vi "addDefectiveRows.vi"(0 "reference in":refnum<class "excelFile.lvclass">, 5 "error in (no error)":errorcluster) -> (14 "reference out":refnum<class "excelFile.lvclass">, 19 "error out":errorcluster)   [LabVIEW 2016, in "excelFile.lvclass"]
uses:
  excelFile.lvclass
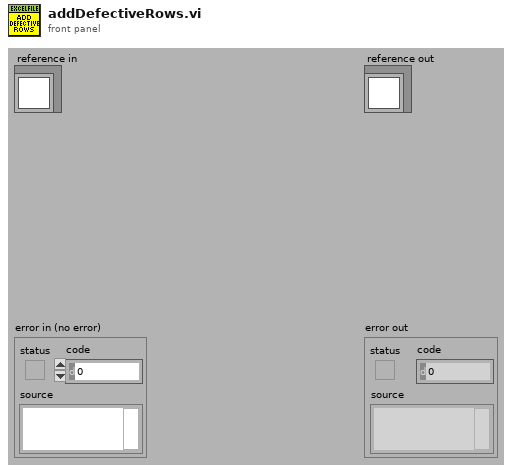
[diagram p1: front panel]
types:
  T1 = typedef "excelFile.lvclass/ObjectAttributesRef.ctl" = refnum<data-value>
  T2 = typedef "excelFile.lvclass/ObjectAttributes.ctl" = cluster{"MyAttribute":dbl, "path":string, "Refnum Excel":cluster{"Excel._Application":refnum<k7>, "Workbooks":refnum<k7>, "Open":refnum<k7>}, "data":string[][][], "save":bool, "fileType":T3, "rowsColor":u32[], "python_ref":refnum<class "python.lvclass">, "items_rows":i32[], "excel_range":i32[][], "TSR":cluster{"number":string, "TSR_path":path, "service_path":path, "email_to":string}, "excel_already_opened?":bool, "file_already_opened?":bool, "excel_protected_opened?":bool, "Refnum Cluster Worksheets":cluster{"Excel._Application":refnum<k7>, "Workbooks":refnum<k7>, "Open":refnum<k7>, "Worksheets":refnum<k7>, "Excel._Worksheet":refnum<k7>}, "#_rows_defective":i32, "#_rows_spare":i32}
  T3 = typedef "excelFile.lvclass/fileType.ctl" = enum16{"devices", "items", "partsTracking", "TSR"}
  T4 = cluster{"Excel._Application":refnum<k7>, "Workbooks":refnum<k7>, "Open":refnum<k7>, "Worksheets":refnum<k7>, "Excel._Worksheet":refnum<k7>}
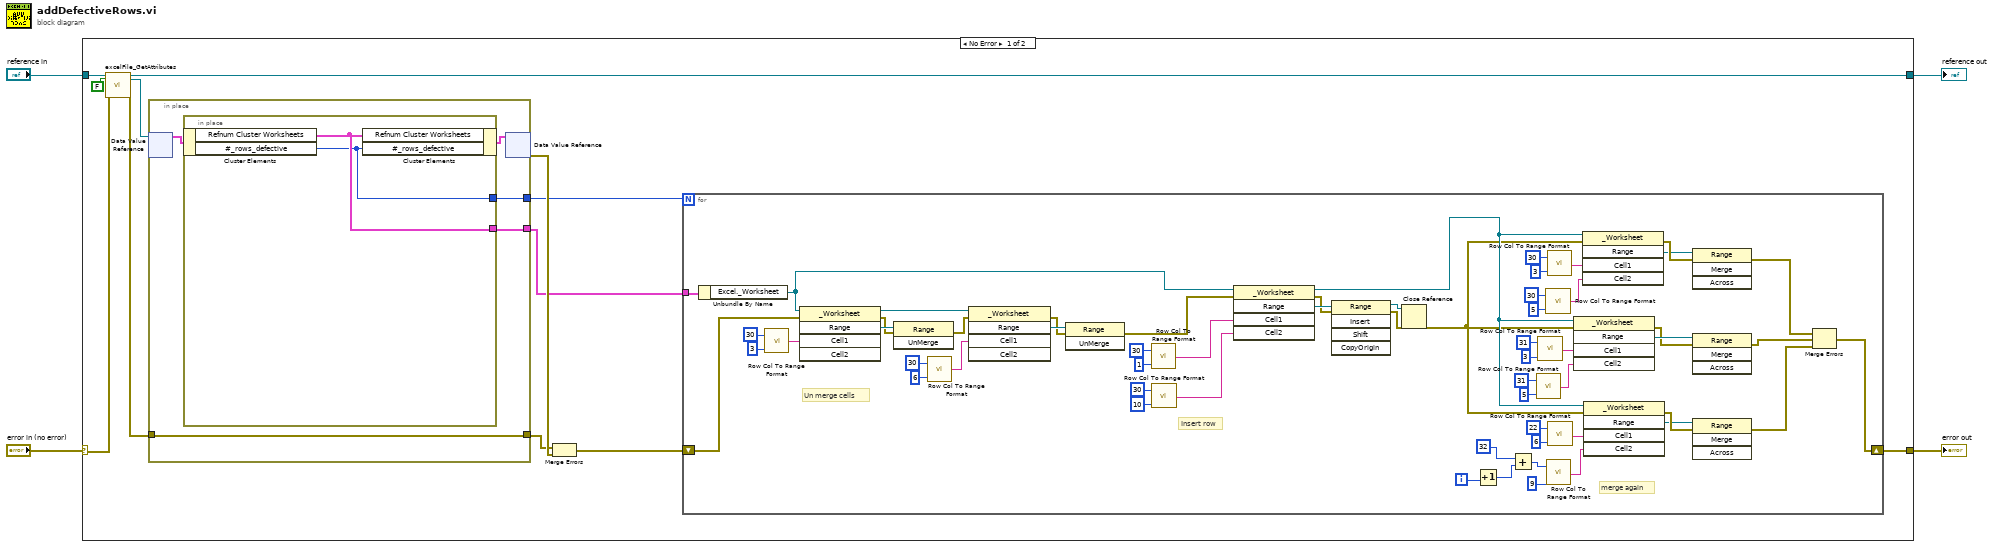
[diagram p0: block diagram]
diagram:
  n1 = case shown="No Error" "error in (no error)" {
    selector: "error in (no error)" -> [w12 w84]
    tunnel: [w6 w84] -> w3
    tunnel: [w10 w83] -> w1
    tunnel: "reference in" -> [w14 w83]
    frame No Error {
      n2 = call "excelFile_GetAttributes.vi"("reference in"=w14, "return data? (T)"=FALSE, "error in (no error)"=w12) -> ("reference out"=w10:refnum<class "excelFile.lvclass">, "attributes ref"=w9:T1, "error out"=w11:errorcluster)  [unwired: 13 in, 1 out]
      n3 = in-place {
        in-place-border: w11 -> [w78]
        in-place-border: [w78] -> w15
        in-place-border: [w77] -> w7
        in-place-border: [w76] -> w5
        n4 = in-place-dvr #1(w9) -> (w79:T2)  [unwired: 1 out]
        n5 = in-place {
          in-place-border: [w82] -> w77
          in-place-border: [w81] -> w76
          n6 = in-place-cluster #2(w79) -> ("Refnum Cluster Worksheets"=w82:T4, "#_rows_defective"=w81:i32)
          n7 = in-place-cluster #2("Refnum Cluster Worksheets"=w82, "#_rows_defective"=w81) -> (w80:T2)
        }
        n8 = in-place-dvr #1(w80) -> (w16:errorcluster)  [unwired: 1 out]
      }
      n9 = Merge Errors(w15, w16) -> (w8:errorcluster)
      n10 = for {
        N: w5 -> [_]
        tunnel: w7 -> [w35]
        shift-right: [w22] -> w6
        shift-left: w8 -> [w36]
        i -> [w19]
        # "merge again"
        # "Insert row"
        # "Un merge cells"
        n11 = Unbundle By Name(w35) -> ("Excel._Worksheet"=w37:refnum<k7>)
        n12 = call <userlib>:"Row Col To Range Format.vi"("Column"=3, "Row"=30) -> ("Output String"=w50:string)
        n13 = invoke class="_Worksheet" method="Range"(reference=w37, error in=w36, "Cell1"=w50) -> (reference out=w42:refnum<k7>, error out=w41:errorcluster, "Range"=w45:refnum<k7>)  [unwired: 2 in, 2 out]
        n14 = invoke class="Range" method="UnMerge"(reference=w45, error in=w41) -> (error out=w40:errorcluster)  [unwired: 1 in, 2 out]
        n15 = call <userlib>:"Row Col To Range Format.vi"("Column"=6, "Row"=30) -> ("Output String"=w47:string)
        n16 = invoke class="_Worksheet" method="Range"(reference=w42, error in=w40, "Cell1"=w47) -> (error out=w39:errorcluster, "Range"=w46:refnum<k7>)  [unwired: 2 in, 3 out]
        n17 = invoke class="Range" method="UnMerge"(reference=w46, error in=w39) -> (error out=w38:errorcluster)  [unwired: 1 in, 2 out]
        n18 = call <userlib>:"Row Col To Range Format.vi"("Column"=1, "Row"=30) -> ("Output String"=w75:string)
        n19 = call <userlib>:"Row Col To Range Format.vi"("Column"=10, "Row"=30) -> ("Output String"=w68:string)
        n20 = invoke class="_Worksheet" method="Range"(reference=w37, error in=w38, "Cell1"=w75, "Cell2"=w68) -> (reference out=w27:refnum<k7>, error out=w53:errorcluster, "Range"=w54:refnum<k7>)  [unwired: 1 in, 2 out]
        n21 = invoke class="Range" method="Insert"(reference=w54, error in=w53) -> (reference out=w72:refnum<k7>, error out=w71:errorcluster)  [unwired: 3 in, 3 out]
        n22 = Close Reference(reference=w72, error in (no error)=w71) -> (error out=w26:errorcluster)
        n23 = Increment(x=w19) -> (x+1=w18:i32)
        n24 = Add(x=32 ("Row"), y=w18) -> (x+y=w21:i32)
        n25 = call <userlib>:"Row Col To Range Format.vi"("Column"=5, "Row"=31) -> ("Output String"=w60:string)
        n26 = call <userlib>:"Row Col To Range Format.vi"("Column"=3, "Row"=31) -> ("Output String"=w65:string)
        n27 = call <userlib>:"Row Col To Range Format.vi"("Column"=5, "Row"=30) -> ("Output String"=w34:string)
        n28 = call <userlib>:"Row Col To Range Format.vi"("Column"=9, "Row"=w21) -> ("Output String"=w43:string)
        n29 = call <userlib>:"Row Col To Range Format.vi"("Column"=3, "Row"=30) -> ("Output String"=w30:string)
        n30 = call <userlib>:"Row Col To Range Format.vi"("Column"=6, "Row"=22) -> ("Output String"=w57:string)
        n31 = invoke class="_Worksheet" method="Range"(reference=w27, error in=w26, "Cell1"=w65, "Cell2"=w60) -> (error out=w63:errorcluster, "Range"=w64:refnum<k7>)  [unwired: 1 in, 3 out]
        n32 = invoke class="_Worksheet" method="Range"(reference=w27, error in=w26, "Cell1"=w30, "Cell2"=w34) -> (error out=w32:errorcluster, "Range"=w31:refnum<k7>)  [unwired: 1 in, 3 out]
        n33 = invoke class="_Worksheet" method="Range"(reference=w27, error in=w26, "Cell1"=w57, "Cell2"=w43) -> (error out=w59:errorcluster, "Range"=w58:refnum<k7>)  [unwired: 1 in, 3 out]
        n34 = invoke class="Range" method="Merge"(reference=w31, error in=w32) -> (error out=w25:errorcluster)  [unwired: 2 in, 3 out]
        n35 = invoke class="Range" method="Merge"(reference=w64, error in=w63) -> (error out=w24:errorcluster)  [unwired: 2 in, 3 out]
        n36 = invoke class="Range" method="Merge"(reference=w58, error in=w59) -> (error out=w23:errorcluster)  [unwired: 2 in, 3 out]
        n37 = Merge Errors(w25, w24, w23) -> (w22:errorcluster)
      }
    }
    frame Error {
    }
  }
  "error out" <- w3
  "reference out" <- w1
